vi "LET Transfer v2.vi"() -> ()   [LabVIEW 2010]
doc: "Cont(inuous) Acq(uire) & Chart (hw timed) demonstrates the hardware timed, non-buffered technique of data acquisition. The scan clock on the board controls acquisition timing. Acquired scans are read directly from the device's FIFO using AI Single Scan. \n\nThe acquisition is configured with no buffer, and the on-board scan clock started at the selected scan rate. In the first loop iteration, the newest (most recent) scan is read from the FIFO. In each subsequent loop iteration AI Single Scan is called to read the oldest scan from the FIFO. Then if a scan is missed because the acquisition does not keep up, an error message will be displayed, and the acquisition stopped. Each scan is plotted on the chart after it is read. \n\nA common reason to use non-buffered acquisition is that some kind of processing needs to be done for each data point. You will probably want to add more functions to the diagram to customize this VI for your application. The acquisition rate you can achieve depends on how much processing and display the VI must do. This VI calls a subVI named My Single-Scan Processing. Add whatever processing you need to this subVI, or replace it with one of your own. The data processing subVI also demonstrates how to use error clusters in your own subVIs, so they can be included in the error data flow chain.\n\nBefore running this VI, set the values of the controls on the front panel. Select Show Help Window from the Help menu to see a description of each control. If the values you select for all the controls are values you will usually use, select Make Current Values Default from the Operate menu and save the VI. Or, you may save individual control's default values by popping up on the control, selecting Data Operations, then selecting Make Current Value Default, and saving the VI."
uses:
  <instrlib>/agilent_b2900_series/Agilent B2900 Series/Public/Configure/Measurement/Configure Measurement (Current).vi
  <instrlib>/agilent_b2900_series/Agilent B2900 Series/Public/Configure/Measurement/Configure Measurement (Voltage).vi
  <vilib>/Utility/file.llb/Write To Spreadsheet File (DBL).vi
  <instrlib>/agilent_b2900_series/Agilent B2900 Series/Agilent B2900 Series.lvlib
panel:
  out "data matrix":dbl[][](array[numeric])
  out "Igs array 2":dbl[][](array[numeric])
  out "Vgs array 2":dbl[][](array[numeric])
  out "Vds array 2":dbl[][](array[numeric])
  out "Corrected PD current array 2":dbl[][](array[numeric])
  out "Ids array 2":dbl[][](array[numeric])
  out "corrected PD current array":dbl[](array[numeric])
  out "Vds array":dbl[](array[numeric])
  out "Ids array":dbl[](array[numeric])
  out "Vgs array":dbl[](array[numeric])
  out "Igs array":dbl[](array[numeric])
  in  "Tab Control":T1(tab)
  in  "keithley address":string="GPIB0::20::INSTR"
  in  "agilent address":refnum<visa-resource-name>="GPIB0::23::INSTR"
  in  "Initial Vgs (V)":sgl format="%.2f"
  in  "Vgs step (V)":sgl=1.0 format="%.2f"
  in  "Vgs delay time (ms)":sgl=10.0 format="%.2f"
  in  "Vgs delay after first value":sgl=10.0 caption="Vgs delay after first value (ms)" format="%.2f"
  in  "Final Vgs(V)":sgl=60.0 format="%.2f"
  in  "light emission ON/OFF":bool=TRUE
  in  "Vds step (V)":sgl=20.0 format="%.2f"
  in  "Final Vds (V)":sgl=60.0 format="%.2f"
  in  "Initial Vds (V)":sgl format="%.2f"
  in  "Vds hold time (ms)":i32=10
  in  "Compliance Voltage (channel 1)":dbl=60.0
  in  "Compliance Current (channel 2)":dbl=0.001
  in  "Compliance Voltage (channel 2)":dbl=60.0
  in  "Compliance Current (channel 1)":dbl=0.0001
  in  "keithley compliance limit":dbl(ring)=0.025 items=["25uA"=2.5e-05, "250uA"=0.00025, "2.5mA"=0.0025, "25mA"=0.025]
  in  "Loop":bool=TRUE
  in  "Auto Current NPLC (F: Disable)":bool
  in  "Auto Voltage NPLC(F: Disable)":bool
  in  "Current NPLC (0.1)":dbl=0.1
  in  "Voltage NPLC (0.1 PLC)":dbl=0.1
  in  "Current Auto Range Mode (0: Normal)":i32(ring) items=["Normal", "Resolution", "Speed"]
  in  "Voltage Auto Range Mode (0: Normal)":i32(ring) items=["Normal", "Resolution", "Speed"]
  in  "aperture time":dbl(ring)=-3.0 format="%.2f" items=["KE6485_VAL_RATE_FAST"=-1.0, "KE6485_VAL_RATE_MEDIUM"=-2.0, "KE6485_VAL_RATE_SLOW"=-3.0]
  in  "resolution (absolute)":dbl=0.0001 format="%^.2e"
  in  "Tab Control 2":enum32{"log scale", "linear scale"}(tab)
  out "Current Scan log":cluster{dbl[], dbl[]}(graph) caption="Current Scan"
  out "Current Scan log2":cluster{dbl[], dbl[]}(graph) caption="Current Scan"
  out "Current Scan linear":cluster{dbl[], dbl[]}(graph) caption="Current Scan"
  out "Current Scan linear 2":cluster{dbl[], dbl[]}(graph) caption="Current Scan"
  out "Applied Vgs":sgl caption="current VDS (V)" format="%.2f"
  out "Applied Vds":sgl caption="current VDS (V)" format="%.2f"
  out "Measured Ids":dbl format="%.2e"
  out "Measured Vds":dbl
  out "corrected PD current":dbl format="%^.2e"
  out "dark PD current (A)":dbl format="%^.2e"
  out "PD current":dbl format="%^.2e"
  out "Measured Igs":dbl
  out "Measured Vgs":dbl
  out "channel 2 status":bool
  out "channel 1 status":bool
  out "half  points":sgl
  out "Vgs points":sgl
  out "Vds points":sgl
  in  "Tab Control 3":enum32{"Log scale", "Linear scale"}(tab)
  out "?":cluster{dbl[], dbl[]}[](graph)
  out "?":cluster{dbl[], dbl[]}[](graph)
  out "?":cluster{dbl[], dbl[]}[](graph)
  out "?":cluster{dbl[], dbl[]}[](graph)
  in  "error in keithley":errorcluster
  out "keithley address out":refnum<k15>
  out "error out keithley":errorcluster
  out "error out agilent":errorcluster
  out "Agilent address out":refnum<visa-resource-name>
  # "LET Transfer v2"
  # "Gate Setting"
  # "Drain-source Setting"
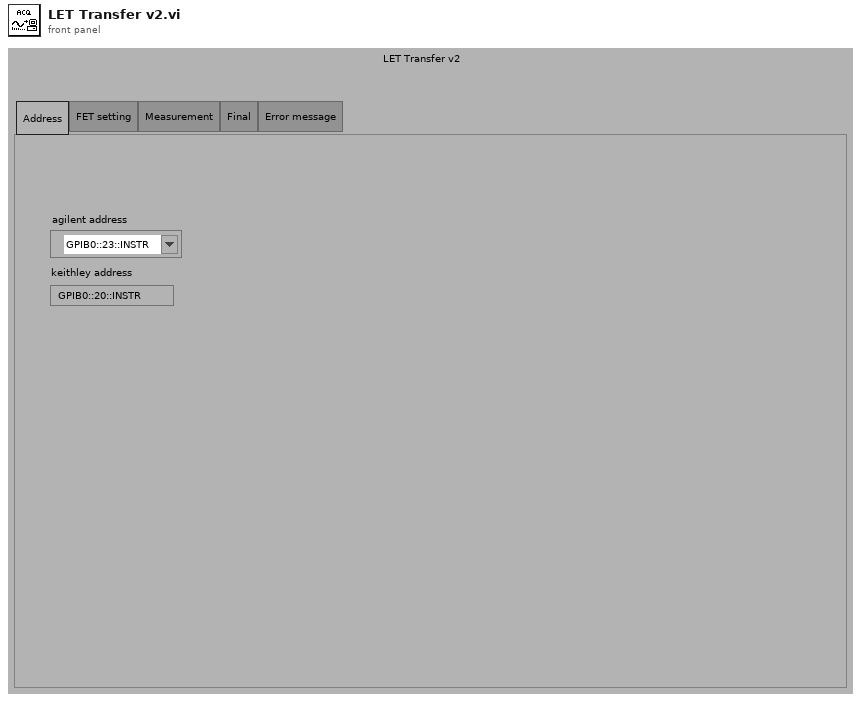
[diagram p1: front panel]
types:
  T1 = enum32{"Address", "FET setting", "Measurement", "Final", "Error message"}
  T2 = typedef "NI_Matrix.lvlib/RealMatrix.ctl" = dbl[][]
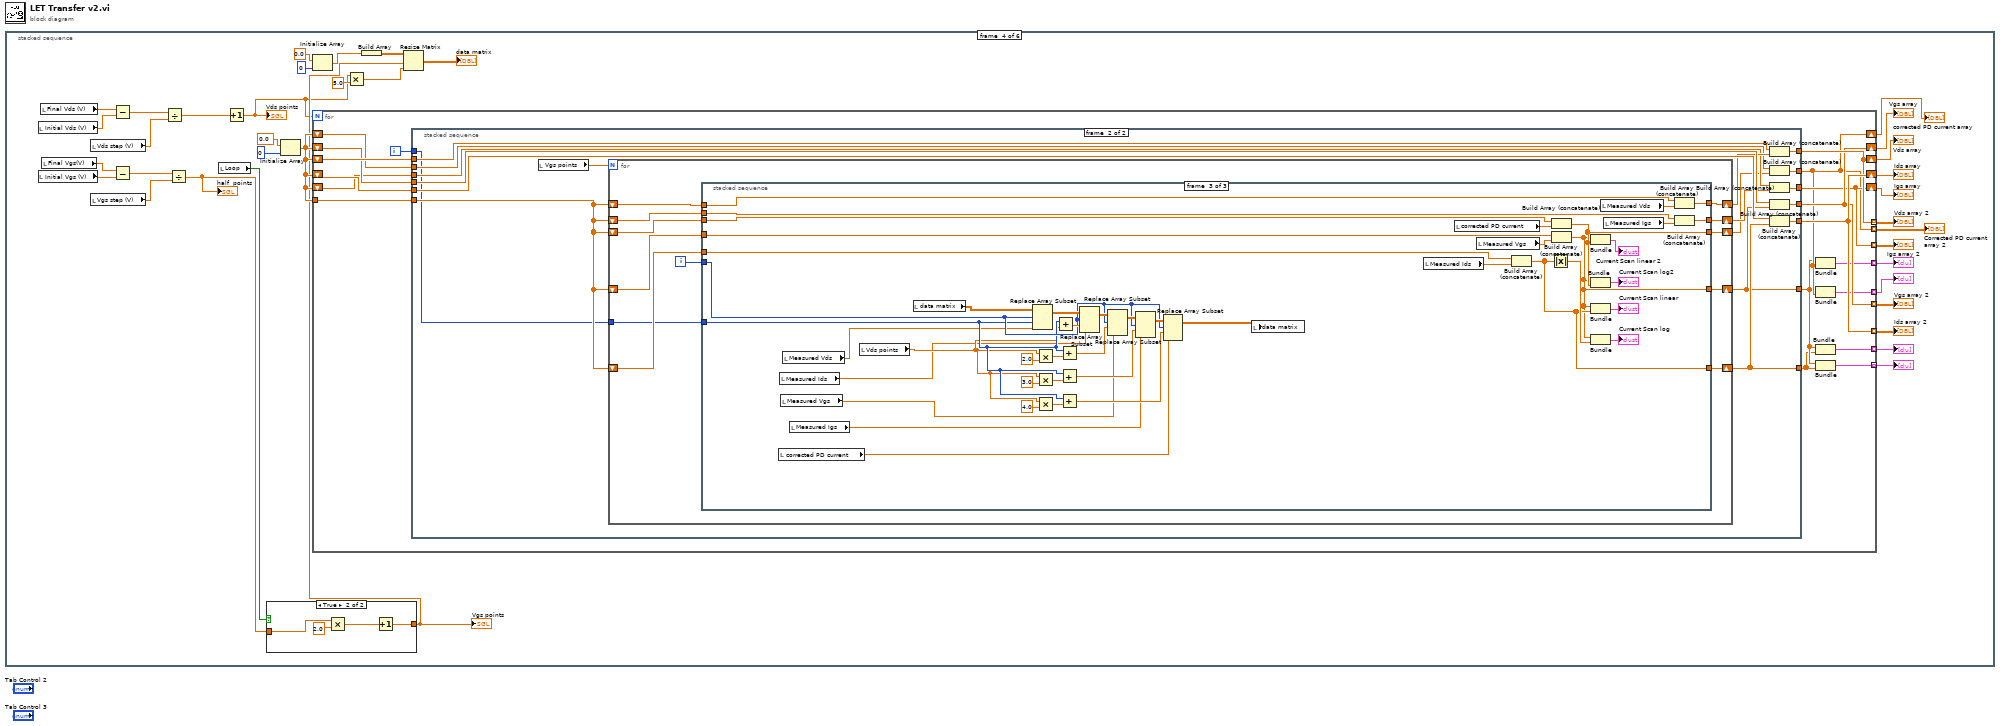
[diagram p0: block diagram]
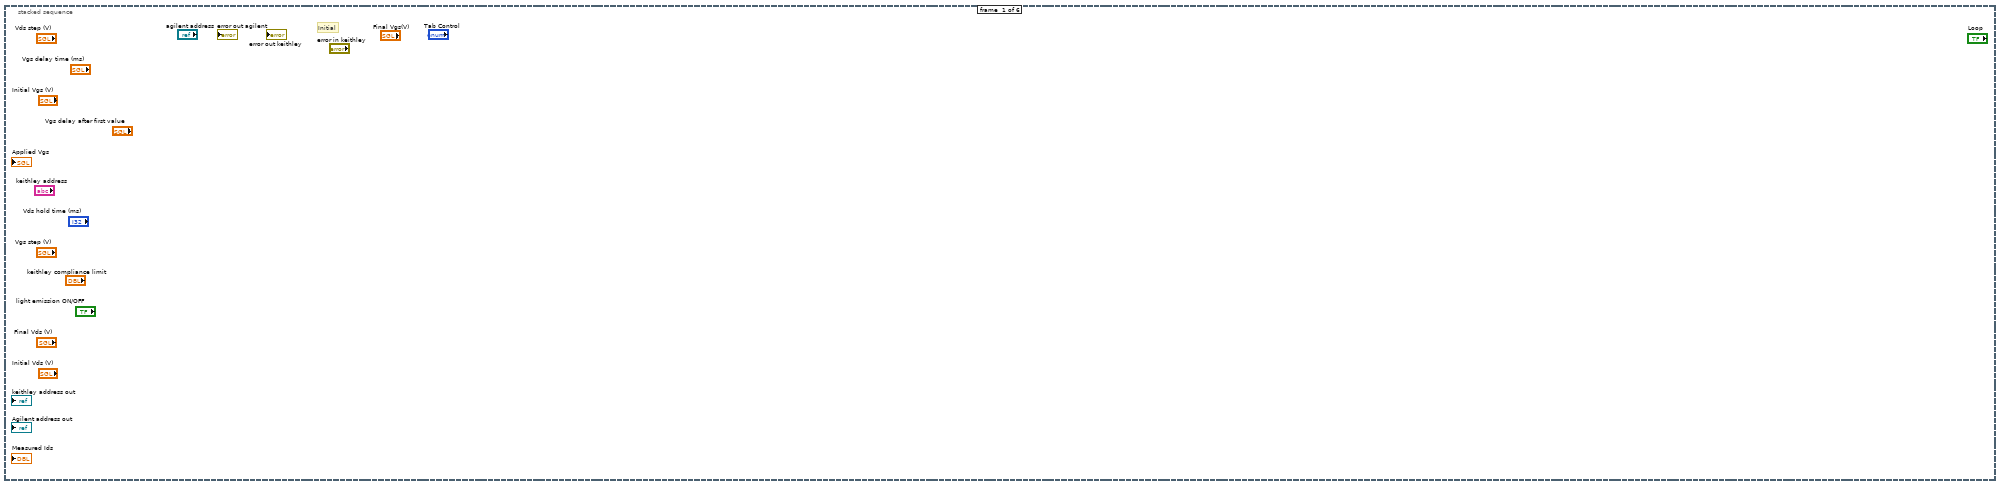
[diagram p2: hidden frame]
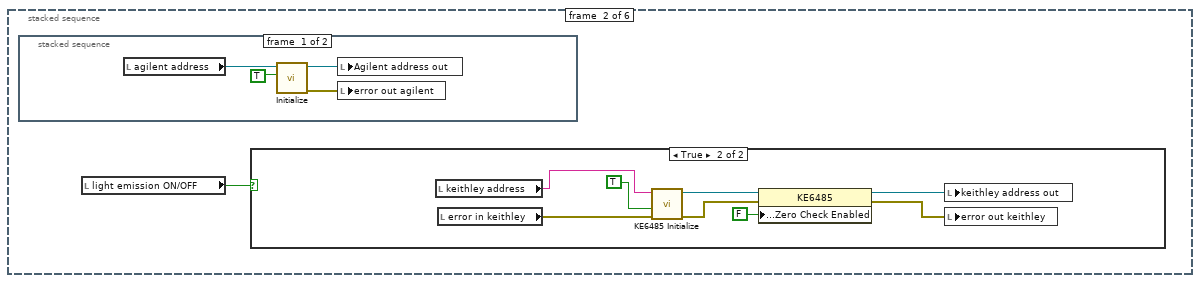
[diagram p3: hidden frame]
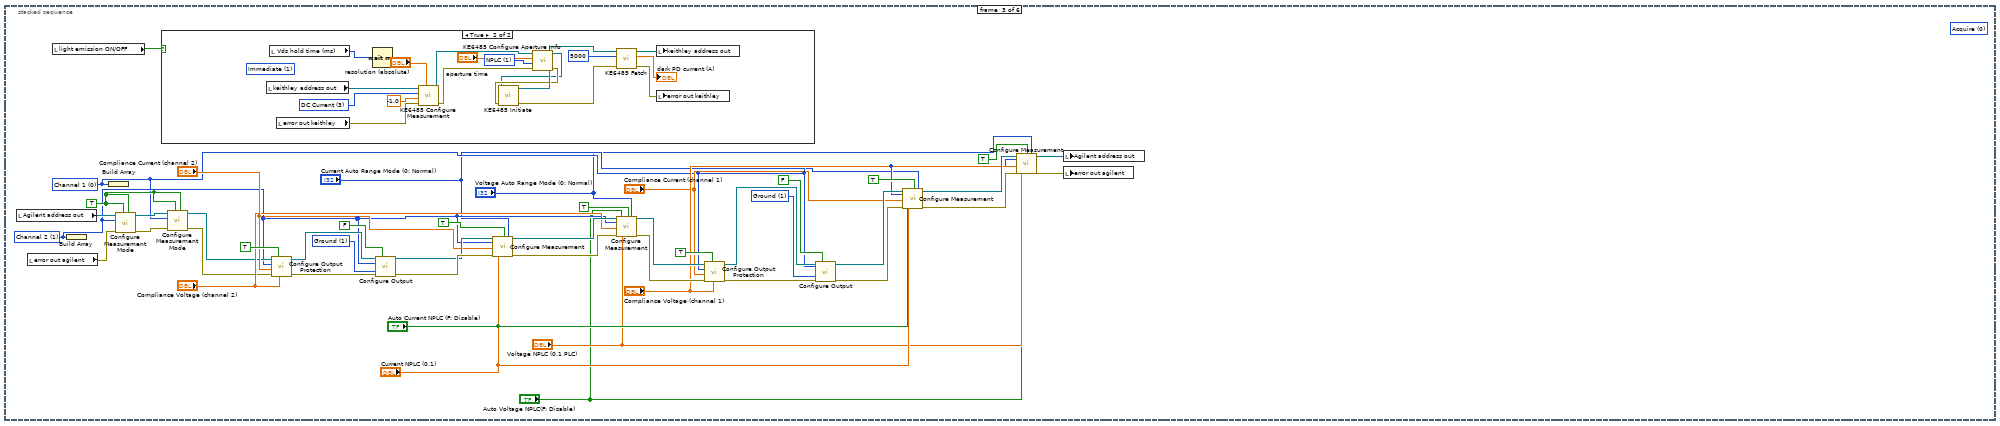
[diagram p6: hidden frame]
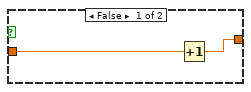
[diagram p8: hidden frame]
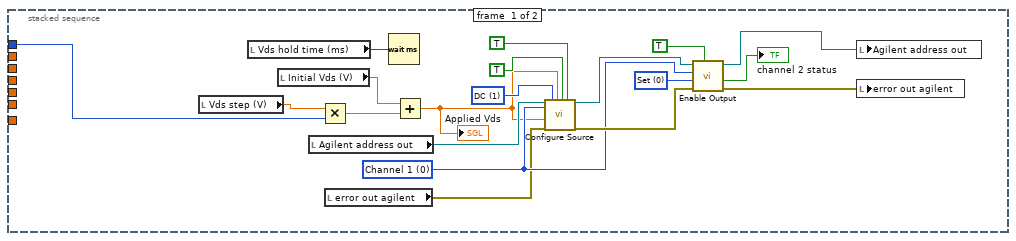
[diagram p9: hidden frame]
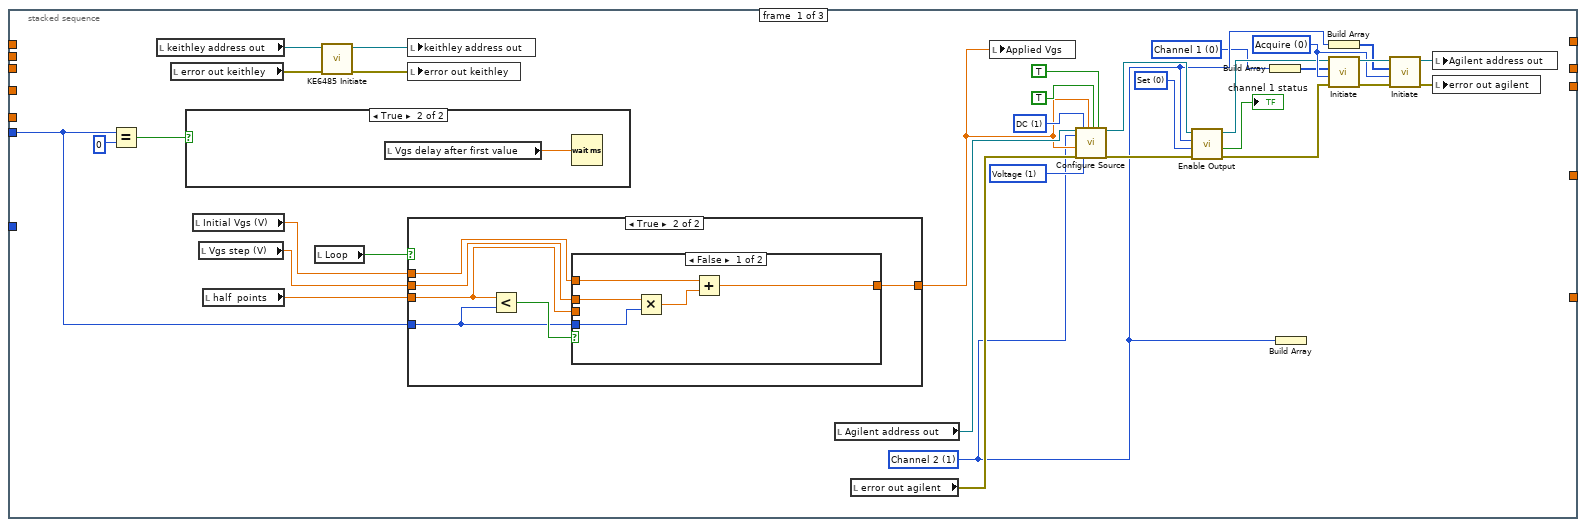
[diagram p10: hidden frame]
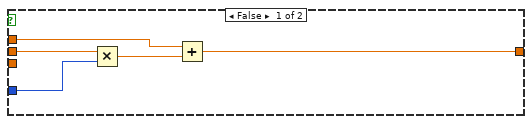
[diagram p11: hidden frame]
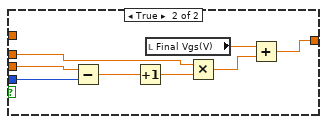
[diagram p12: hidden frame]
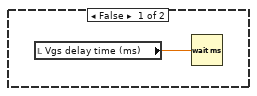
[diagram p13: hidden frame]
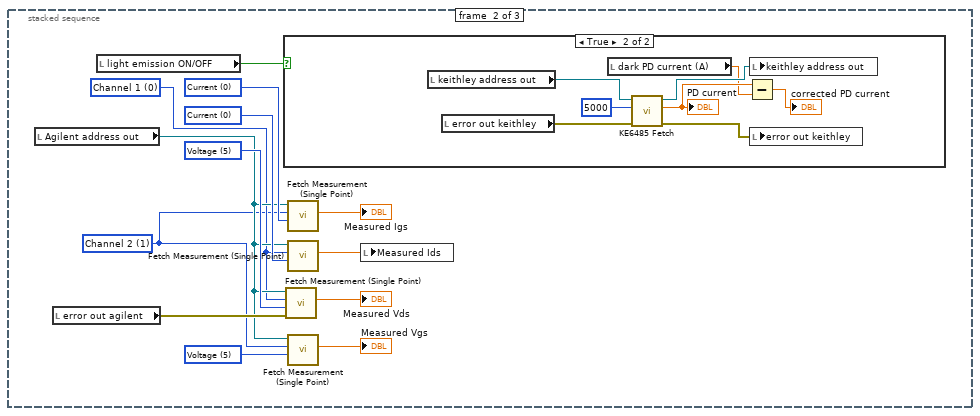
[diagram p14: hidden frame]
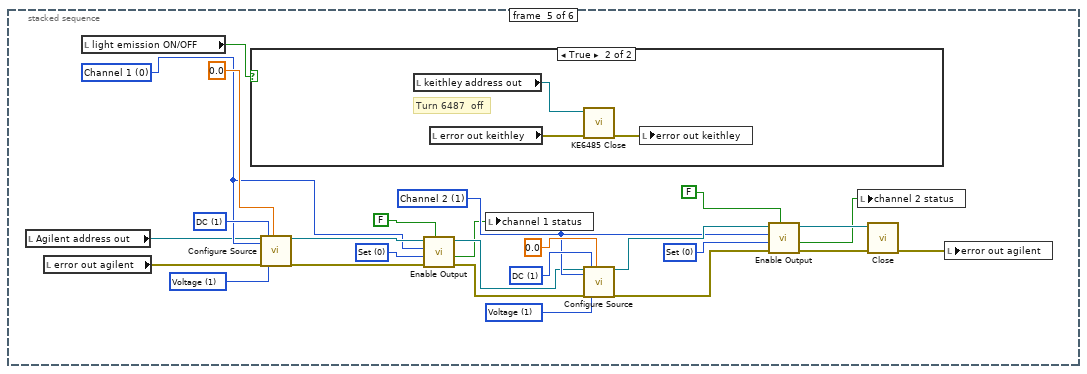
[diagram p16: hidden frame]
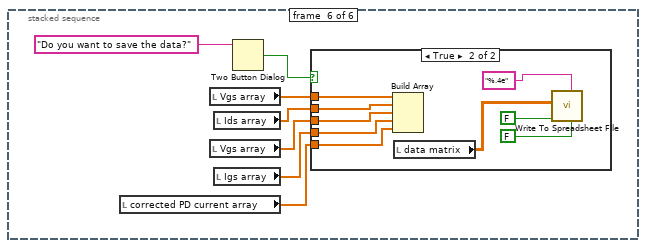
[diagram p18: hidden frame]
diagram:
  n1 = stacked-sequence {
    frame #0 {
      # "Initial"
    }
    frame #1 {
      n2 = stacked-sequence {
        frame #0 {
          n3 = local read "agilent address"() -> (w2:refnum<visa-resource-name>)
          n4 = call <instrlib>:"Initialize.vi"("ID Query (True)"=TRUE, "VISA resource name"=w2) -> ("error out"=w3:errorcluster, "VISA resource name out"=w4:refnum<visa-resource-name>)  [unwired: 8 in]
          n5 = local write "Agilent address out"(w4) -> ()
          n6 = local write "error out agilent"(w3) -> ()
        }
        frame #1 {
        }
      }
      n7 = local read "light emission ON/OFF"() -> (w1:bool)
      n8 = case shown="True" w1 {
        frame False {
        }
        frame True {
          n9 = local read "keithley address"() -> (w12:string)
          n10 = local read "error in keithley"() -> (w13:errorcluster)
          n11 = call <instrlib>:"KE6485 Initialize.vi"("error in (no error)"=w13, "reset device"=TRUE, "resource name"=w12) -> ("error out"=w10:errorcluster, "instrument handle out"=w9:refnum<k15>)  [unwired: 1 in, 6 out]
          n12 = property class="KE6485"(reference=w9, error in=w10, "System Settings:Zero Check Enabled"=FALSE) -> (reference out=w8:refnum<k15>, error out=w7:errorcluster)
          n13 = local write "keithley address out"(w8) -> ()
          n14 = local write "error out keithley"(w7) -> ()
        }
      }
    }
    frame #2 {
      (unwired) 0 items=["Acquire", "Transient", "Both"] ("Device Action (2: Both)")
      w30 = TRUE ("Enable Voltage Measurement (T: Enable)")
      w42 = 1 items=["Float", "Ground"] ("Low Terminal State (1: Ground)")
      w22 = 0 items=["Channel 1", "Channel 2"] ("Channel (0: Channel 1)")
      w52 = 1 items=["Float", "Ground"] ("Low Terminal State (1: Ground)")
      w23 = 1 items=["Channel 1", "Channel 2"] ("Channel (0: Channel 1)")
      n15 = local read "Agilent address out"() -> (w25:refnum<visa-resource-name>)
      n16 = local read "error out agilent"() -> (w27:errorcluster)
      n17 = local read "light emission ON/OFF"() -> (w59:bool)
      n18 = Build Array(w23) -> ()  [unwired: 1 out]
      n19 = Build Array(w22) -> ()  [unwired: 1 out]
      n20 = call <instrlib>:"Configure Measurement Mode.vi"("Enable Current Measurement (T: Enable)"=w30, "Enable Voltage Measurement (T: Enable)"=w30, "error in (no error)"=w27, "Channel (0: Channel 1)"=w23, "VISA resource name"=w25) -> ("error out"=w28:errorcluster, "VISA resource name out"=w29:refnum<visa-resource-name>)  [unwired: 5 in]
      n21 = case shown="True" w59 {
        frame False {
        }
        frame True {
          w66 = 1 items=["NPLC"=1] ("aperture time unit")
          (unwired) 1 items=["Immediate"=1, "Interval"=10, "Trigger Link 1"=1001, "Trigger Link 2"=1002, "Trigger Link 3"=1003, "Trigger Link 4"=1004, "Trigger Link 5"=1005, "Trigger Link 6"=1006] ("sample trigger")
          w75 = 3 items=["DC Volts"=1, "DC Current"=3, "2 Wire Resistance"=5, "Charge"=1004] ("measurement function")
          n22 = local read "keithley address out"() -> (w70:refnum<k15>)
          n23 = local read "Vds hold time (ms)"() -> (w77:i32)
          n24 = local read "error out keithley"() -> (w69:errorcluster)
          n25 = Wait (ms)(milliseconds to wait=w77) -> ()  [unwired: 1 out]
          n26 = call <instrlib>:"KE6485 Configure Measurement.vi"("resolution (absolute)"="resolution (absolute)", "error in (no error)"=w69, "range"=-1.0, "measurement function"=w75, "instrument handle"=w70) -> ("error out"=w65:errorcluster, "instrument handle out"=w64:refnum<k15>)  [unwired: 5 in]
          n27 = call <instrlib>:"KE6485 Configure Aperture Info.vi"("error in (no error)"=w65, "aperture time unit"=w66, "aperture time"="aperture time", "instrument handle"=w64) -> ("error out"=w63:errorcluster, "instrument handle out"=w62:refnum<k15>)  [unwired: 6 in]
          n28 = call <instrlib>:"KE6485 Initiate.vi"("error in (no error)"=w63, "instrument handle"=w62) -> ("error out"=w67:errorcluster, "instrument handle out"=w68:refnum<k15>)  [unwired: 8 in]
          n29 = call <instrlib>:"KE6485 Fetch.vi"("error in (no error)"=w67, "maximum time (ms)"=5000, "instrument handle"=w68) -> ("error out"=w72:errorcluster, "reading"=→"dark PD current (A)":dbl, "instrument handle out"=w71:refnum<k15>)  [unwired: 6 in]
          n30 = local write "keithley address out"(w71) -> ()
          n31 = local write "error out keithley"(w72) -> ()
        }
      }
      n32 = call <instrlib>:"Configure Measurement Mode.vi"("Enable Current Measurement (T: Enable)"=w30, "Enable Voltage Measurement (T: Enable)"=w30, "error in (no error)"=w28, "Channel (0: Channel 1)"=w22, "VISA resource name"=w29) -> ("error out"=w26:errorcluster, "VISA resource name out"=w24:refnum<visa-resource-name>)  [unwired: 5 in]
      n33 = call <instrlib>:"Configure Output Protection.vi"("Compliance Voltage (2 V)"="Compliance Voltage (channel 2)", "Enable Output Protection (T: Enable)"=TRUE, "error in (no error)"=w26, "Compliance Current (0.0001 A)"="Compliance Current (channel 2)", "Channel (0: Channel 1)"=w23, "VISA resource name"=w24) -> ("error out"=w54:errorcluster, "VISA resource name out"=w53:refnum<visa-resource-name>)  [unwired: 4 in]
      n34 = call <instrlib>:"Configure Output.vi"("VISA resource name"=w53, "Auto Output-Off (F: Disable)"=FALSE, "Channel (0: Channel 1)"=w23, "Low Terminal State (1: Ground)"=w52, "error in (no error)"=w54) -> ("VISA resource name out"=w50:refnum<visa-resource-name>, "error out"=w51:errorcluster)  [unwired: 9 in]
      n35 = call-poly <instrlib>:"Configure Measurement.vi"("VISA resource name"=w50, "Channel (0: Channel 1)"=w23, "Current Range (0.0001 A)"="Compliance Current (channel 2)", "error in (no error)"=w51, "Auto Current NPLC (F: Disable)"="Auto Current NPLC (F: Disable)", "Current NPLC (0.1)"="Current NPLC (0.1)", "Current Auto Range (T: Enable)"=TRUE, "Current Auto Range Mode (0: Normal)"="Current Auto Range Mode (0: Normal)") -> ("VISA resource name out"=w58:refnum<visa-resource-name>, "error out"=w57:errorcluster)  [unwired: 10 in]
      n36 = call-poly <instrlib>:"Configure Measurement.vi"("VISA resource name"=w58, "Channel (0: Channel 1)"=w23, "Voltage Range (2 V)"="Compliance Voltage (channel 2)", "error in (no error)"=w57, "Auto Voltage NPLC(F: Disable)"="Auto Voltage NPLC(F: Disable)", "Voltage NPLC (0.1 PLC)"="Voltage NPLC (0.1 PLC)", "Voltage Auto Range (T: Enable)"=TRUE, "Voltage Auto Range Mode (0: Normal)"="Voltage Auto Range Mode (0: Normal)") -> ("VISA resource name out"=w38:refnum<visa-resource-name>, "error out"=w37:errorcluster)  [unwired: 10 in]
      n37 = call <instrlib>:"Configure Output Protection.vi"("Compliance Voltage (2 V)"="Compliance Voltage (channel 1)", "Enable Output Protection (T: Enable)"=TRUE, "error in (no error)"=w37, "Compliance Current (0.0001 A)"="Compliance Current (channel 1)", "Channel (0: Channel 1)"=w22, "VISA resource name"=w38) -> ("error out"=w44:errorcluster, "VISA resource name out"=w43:refnum<visa-resource-name>)  [unwired: 4 in]
      n38 = call <instrlib>:"Configure Output.vi"("VISA resource name"=w43, "Auto Output-Off (F: Disable)"=FALSE, "Channel (0: Channel 1)"=w22, "Low Terminal State (1: Ground)"=w42, "error in (no error)"=w44) -> ("VISA resource name out"=w40:refnum<visa-resource-name>, "error out"=w41:errorcluster)  [unwired: 9 in]
      n39 = call-poly <instrlib>:"Configure Measurement.vi"("VISA resource name"=w40, "Channel (0: Channel 1)"=w22, "Current Range (0.0001 A)"="Compliance Current (channel 1)", "error in (no error)"=w41, "Auto Current NPLC (F: Disable)"="Auto Current NPLC (F: Disable)", "Current NPLC (0.1)"="Current NPLC (0.1)", "Current Auto Range (T: Enable)"=TRUE, "Current Auto Range Mode (0: Normal)"="Current Auto Range Mode (0: Normal)") -> ("VISA resource name out"=w48:refnum<visa-resource-name>, "error out"=w47:errorcluster)  [unwired: 10 in]
      n40 = call-poly <instrlib>:"Configure Measurement.vi"("VISA resource name"=w48, "Channel (0: Channel 1)"=w22, "Voltage Range (2 V)"="Compliance Voltage (channel 1)", "error in (no error)"=w47, "Auto Voltage NPLC(F: Disable)"="Auto Voltage NPLC(F: Disable)", "Voltage NPLC (0.1 PLC)"="Voltage NPLC (0.1 PLC)", "Voltage Auto Range (T: Enable)"=TRUE, "Voltage Auto Range Mode (0: Normal)"="Voltage Auto Range Mode (0: Normal)") -> ("VISA resource name out"=w21:refnum<visa-resource-name>, "error out"=w20:errorcluster)  [unwired: 10 in]
      n41 = local write "Agilent address out"(w21) -> ()
      n42 = local write "error out agilent"(w20) -> ()
    }
    frame #3 {
      n43 = local read "Initial Vds (V)"() -> (w103:sgl)
      n44 = local read "Initial Vgs (V)"() -> (w106:sgl)
      n45 = local read "Final Vds (V)"() -> (w102:sgl)
      n46 = local read "Final Vgs(V)"() -> (w105:sgl)
      n47 = local read "Vds step (V)"() -> (w104:sgl)
      n48 = local read "Vgs step (V)"() -> (w107:sgl)
      n49 = Subtract(x=w102, y=w103) -> (x-y=w100:sgl)
      n50 = Subtract(x=w105, y=w106) -> (x-y=w114:sgl)
      n51 = Divide(x=w100, y=w104) -> (x/y=w101:sgl)
      n52 = Divide(x=w114, y=w107) -> (x/y=w98:sgl)
      "half  points" <- w98
      n53 = local read "Loop"() -> (w99:bool)
      n54 = Increment(x=w101) -> (x+1=w78:sgl)
      "Vds points" <- w78
      n55 = case shown="True" w99 {
        tunnel: w98 -> [w116 w120]
        tunnel: [w115 w118] -> w81
        frame False {
          n56 = Increment(x=w116) -> (x+1=w115:sgl)
        }
        frame True {
          n57 = Multiply(x=w120, y=sgl 2.0) -> (x*y=w117:sgl)
          n58 = Increment(x=w117) -> (x+1=w118:sgl)
        }
      }
      "Vgs points" <- w81
      n59 = Initialize Array(0.0, 0) -> (w95:dbl[])
      n60 = Initialize Array(0.0 ("element"), 0 ("dimension size")) -> (w84:dbl[])
      n61 = for {
        N: w78 -> [_]
        shift-right: [w129] -> w110
        shift-left: w95 -> [w137]
        shift-right: [w130] -> w111
        shift-left: w95 -> [w136]
        shift-right: [w128] -> w109
        shift-left: w95 -> [w135]
        tunnel: [w134] -> w108 mode=indexing
        shift-right: [w127] -> w97
        shift-left: w95 -> [w133]
        shift-right: [w125] -> w96
        shift-left: w95 -> [w132]
        tunnel: w95 -> [w131]
        tunnel: [w130] -> w94 mode=indexing
        tunnel: [w125] -> w93 mode=indexing
        tunnel: [w129] -> w92 mode=indexing
        tunnel: [w128] -> w91 mode=indexing
        tunnel: [w127] -> w90 mode=indexing
        tunnel: [w126] -> w89 mode=indexing
        tunnel: [w124] -> w88 mode=indexing
        tunnel: [w121] -> w87 mode=indexing
        i -> [w138]
        n62 = stacked-sequence {
          tunnel: w138 -> [w153 w158]
          tunnel: w137 -> [_ w175]
          tunnel: w136 -> [_ w174]
          tunnel: [_ w170] -> w129
          tunnel: [_ w173] -> w130
          tunnel: w135 -> [_ w172]
          tunnel: [_ w171] -> w128
          tunnel: [_ w159] -> w123
          tunnel: [_ w168] -> w122
          tunnel: w133 -> [_ w167]
          tunnel: [_ w166] -> w127
          tunnel: [_ w164] -> w125
          tunnel: w132 -> [_ w162]
          tunnel: w131 -> [_ w160]
          frame #0 {
            w146 = 0 items=["Set", "Get"] ("Operation (0: Set)")
            w147 = 0 items=["Channel 1", "Channel 2"] ("Channel (0: Channel 1)")
            w150 = 1 items=["Pulse", "DC"] ("Source Shape (1: DC)")
            n63 = local read "Vds step (V)"() -> (w157:sgl)
            n64 = local read "Vds hold time (ms)"() -> (w155:i32)
            n65 = local read "Initial Vds (V)"() -> (w156:sgl)
            n66 = local read "Agilent address out"() -> (w143:refnum<visa-resource-name>)
            n67 = Multiply(x=w157, y=w153) -> (x*y=w154:sgl)
            n68 = local read "error out agilent"() -> (w142:errorcluster)
            n69 = Wait (ms)(milliseconds to wait=w155) -> ()  [unwired: 1 out]
            n70 = Add(x=w156, y=w154) -> (x+y=w139:sgl)
            "Applied Vds" <- w139
            n71 = call <instrlib>:"Configure Source.vi"("VISA resource name"=w143, "Channel (0: Channel 1)"=w147, "Source Range (2)"=w139, "error in (no error)"=w142, "Source Shape (1: DC)"=w150, "Output Level (0)"=w139, "Source Auto Range (T: Enable)"=TRUE, "Enable Continuous Output (T: Enable)"=TRUE) -> ("VISA resource name out"=w152:refnum<visa-resource-name>, "error out"=w151:errorcluster)  [unwired: 10 in]
            n72 = call <instrlib>:"Enable Output.vi"("Enable Output (T: Enable)"=TRUE, "error in (no error)"=w151, "Operation (0: Set)"=w146, "Channel (0: Channel 1)"=w147, "VISA resource name"=w152) -> ("error out"=w141:errorcluster, "Output Enabled?"=→"channel 2 status":bool, "VISA resource name out"=w140:refnum<visa-resource-name>)  [unwired: 4 in]
            n73 = local write "Agilent address out"(w140) -> ()
            n74 = local write "error out agilent"(w141) -> ()
          }
          frame #1 {
            n75 = local read "Vgs points"() -> (w161:sgl)
            n76 = for {
              N: w161 -> [_]
              shift-right: [w178] -> w168
              shift-left: w160 -> [w177]
              shift-right: [w180] -> w169
              shift-left: w160 -> [w179]
              shift-right: [w184] -> w159
              shift-left: w160 -> [w183]
              shift-right: [w182] -> w165
              shift-left: w160 -> [w181]
              shift-right: [w185] -> w163
              shift-left: w160 -> [w186]
              tunnel: w158 -> [w176]
              i -> [w187]
              n77 = stacked-sequence {
                tunnel: w187 -> [w207 _ w276]
                tunnel: w186 -> [_ _ w310]
                tunnel: [_ _ w295] -> w185
                tunnel: [_ _ w292] -> w184
                tunnel: w183 -> [_ _ w308]
                tunnel: [_ _ w294] -> w182
                tunnel: w181 -> [_ _ w306]
                tunnel: [_ _ w299] -> w180
                tunnel: w179 -> [_ _ w303]
                tunnel: [_ _ w293] -> w178
                tunnel: w177 -> [_ _ w301]
                tunnel: w176 -> [_ _ w275]
                frame #0 {
                  w200 = 0 items=["Acquire", "Transient", "Both"] ("Device Action (2: Both)")
                  w192 = 0 items=["Channel 1", "Channel 2"] ("Channel (0: Channel 1)")
                  w209 = 1 items=["Current", "Voltage"] ("Source Mode (1: Voltage)")
                  w212 = 1 items=["Pulse", "DC"] ("Source Shape (1: DC)")
                  w193 = 1 items=["Channel 1", "Channel 2"] ("Channel (0: Channel 1)")
                  w216 = 0 items=["Set", "Get"] ("Operation (0: Set)")
                  n78 = Equal?(x=w207, y=0) -> (x = y?=w219:bool)
                  n79 = local read "keithley address out"() -> (w189:refnum<k15>)
                  n80 = local read "error out keithley"() -> (w188:errorcluster)
                  n81 = case shown="True" w219 {
                    frame False {
                      n82 = local read "Vgs delay time (ms)"() -> (w245:sgl)
                      n83 = Wait (ms)(milliseconds to wait=w245) -> ()  [unwired: 1 out]
                    }
                    frame True {
                      n84 = local read "Vgs delay after first value"() -> (w246:sgl)
                      n85 = Wait (ms)(milliseconds to wait=w246) -> ()  [unwired: 1 out]
                    }
                  }
                  n86 = local read "Initial Vgs (V)"() -> (w208:sgl)
                  n87 = local read "Vgs step (V)"() -> (w206:sgl)
                  n88 = local read "half  points"() -> (w204:sgl)
                  n89 = local read "Loop"() -> (w205:bool)
                  n90 = call <instrlib>:"KE6485 Initiate.vi"("error in (no error)"=w188, "instrument handle"=w189) -> ("error out"=w191:errorcluster, "instrument handle out"=w190:refnum<k15>)  [unwired: 8 in]
                  n91 = local write "keithley address out"(w190) -> ()
                  n92 = local write "error out keithley"(w191) -> ()
                  n93 = case shown="True" w205 {
                    tunnel: [w224 w230] -> w203
                    tunnel: w207 -> [w223 w227]
                    tunnel: w208 -> [w222 w229]
                    tunnel: w206 -> [w221 w228]
                    tunnel: w204 -> [_ w226]
                    frame False {
                      n94 = Multiply(x=w221, y=w223) -> (x*y=w225:sgl)
                      n95 = Add(x=w222, y=w225) -> (x+y=w224:sgl)
                    }
                    frame True {
                      n96 = Less?(x=w226, y=w227) -> (x < y?=w231:bool)
                      n97 = case shown="False" w231 {
                        tunnel: [w235 w244] -> w230
                        tunnel: w229 -> [w234 _]
                        tunnel: w227 -> [w233 w241]
                        tunnel: w228 -> [w232 w242]
                        tunnel: w226 -> [_ w240]
                        frame False {
                          n98 = Multiply(x=w232, y=w233) -> (x*y=w236:sgl)
                          n99 = Add(x=w234, y=w236) -> (x+y=w235:sgl)
                        }
                        frame True {
                          n100 = Subtract(x=w240, y=w241) -> (x-y=w238:sgl)
                          n101 = Increment(x=w238) -> (x+1=w237:sgl)
                          n102 = local read "Final Vgs(V)"() -> (w239:sgl)
                          n103 = Multiply(x=w242, y=w237) -> (x*y=w243:sgl)
                          n104 = Add(x=w239, y=w243) -> (x+y=w244:sgl)
                        }
                      }
                    }
                  }
                  n105 = local read "Agilent address out"() -> (w214:refnum<visa-resource-name>)
                  n106 = local read "error out agilent"() -> (w213:errorcluster)
                  n107 = local write "Applied Vgs"(w203) -> ()
                  n108 = call <instrlib>:"Configure Source.vi"("VISA resource name"=w214, "Channel (0: Channel 1)"=w193, "Source Range (2)"=w203, "error in (no error)"=w213, "Source Shape (1: DC)"=w212, "Source Mode (1: Voltage)"=w209, "Output Level (0)"=w203, "Source Auto Range (T: Enable)"=TRUE, "Enable Continuous Output (T: Enable)"=TRUE) -> ("VISA resource name out"=w218:refnum<visa-resource-name>, "error out"=w217:errorcluster)  [unwired: 9 in]
                  n109 = call <instrlib>:"Enable Output.vi"("error in (no error)"=w217, "Operation (0: Set)"=w216, "Channel (0: Channel 1)"=w193, "VISA resource name"=w218) -> ("error out"=w196:errorcluster, "Output Enabled?"=→"channel 1 status":bool, "VISA resource name out"=w197:refnum<visa-resource-name>)  [unwired: 5 in]
                  n110 = Build Array(w192) -> (w199:i32[])
                  n111 = Build Array(w193) -> ()  [unwired: 1 out]
                  n112 = Build Array(w193) -> (w198:i32[])
                  n113 = call <instrlib>:"Initiate.vi"("error in (no error)"=w196, "Device Action (2: Both)"=w200, "Channel List ({Channel1})"=w199, "VISA resource name"=w197) -> ("error out"=w202:errorcluster, "VISA resource name out"=w201:refnum<visa-resource-name>)  [unwired: 6 in]
                  n114 = call <instrlib>:"Initiate.vi"("error in (no error)"=w202, "Device Action (2: Both)"=w200, "Channel List ({Channel1})"=w198, "VISA resource name"=w201) -> ("error out"=w195:errorcluster, "VISA resource name out"=w194:refnum<visa-resource-name>)  [unwired: 6 in]
                  n115 = local write "Agilent address out"(w194) -> ()
                  n116 = local write "error out agilent"(w195) -> ()
                }
                frame #1 {
                  w248 = 1 items=["Channel 1", "Channel 2"] ("Channel (0: Channel 1)")
                  w249 = 0 items=["Channel 1", "Channel 2"] ("Channel (0: Channel 1)")
                  w254 = 0 items=["Current", "Resistance", "Source Output Setting", "Status", "Time", "Voltage"] ("Data Mode (5: Voltage)")
                  w255 = 5 items=["Current", "Resistance", "Source Output Setting", "Status", "Time", "Voltage"] ("Data Mode (5: Voltage)")
                  w257 = 0 items=["Current", "Resistance", "Source Output Setting", "Status", "Time", "Voltage"] ("Data Mode (5: Voltage)")
                  w259 = 5 items=["Current", "Resistance", "Source Output Setting", "Status", "Time", "Voltage"] ("Data Mode (5: Voltage)")
                  n117 = local read "Agilent address out"() -> (w250:refnum<visa-resource-name>)
                  n118 = local read "error out agilent"() -> (w251:errorcluster)
                  n119 = local read "light emission ON/OFF"() -> (w247:bool)
                  n120 = case shown="True" w247 {
                    frame False {
                    }
                    frame True {
                      n121 = local read "keithley address out"() -> (w261:refnum<k15>)
                      n122 = local read "error out keithley"() -> (w260:errorcluster)
                      n123 = local read "dark PD current (A)"() -> (w262:dbl)
                      n124 = call <instrlib>:"KE6485 Fetch.vi"("error in (no error)"=w260, "maximum time (ms)"=5000, "instrument handle"=w261) -> ("error out"=w266:errorcluster, "reading"=w263:dbl, "instrument handle out"=w265:refnum<k15>)  [unwired: 6 in]
                      "PD current" <- w263
                      n125 = Subtract(x=w263, y=w262) -> (x-y=→"corrected PD current":dbl)
                      n126 = local write "keithley address out"(w265) -> ()
                      n127 = local write "error out keithley"(w266) -> ()
                    }
                  }
                  n128 = call <instrlib>:"Fetch Measurement (Single Point).vi"("error in (no error)"=w251, "Data Mode (5: Voltage)"=w259, "Channel (0: Channel 1)"=w249, "VISA resource name"=w250) -> ("Measurement"=→"Measured Vds":dbl)  [unwired: 5 in, 2 out]
                  n129 = call <instrlib>:"Fetch Measurement (Single Point).vi"("Data Mode (5: Voltage)"=w254, "Channel (0: Channel 1)"=w248, "VISA resource name"=w250) -> ("Measurement"=→"Measured Igs":dbl)  [unwired: 6 in, 2 out]
                  n130 = call <instrlib>:"Fetch Measurement (Single Point).vi"("Data Mode (5: Voltage)"=w257, "Channel (0: Channel 1)"=w249, "VISA resource name"=w250) -> ("Measurement"=w256:dbl)  [unwired: 6 in, 2 out]
                  n131 = call <instrlib>:"Fetch Measurement (Single Point).vi"("Data Mode (5: Voltage)"=w255, "Channel (0: Channel 1)"=w248, "VISA resource name"=w250) -> ("Measurement"=→"Measured Vgs":dbl)  [unwired: 6 in, 2 out]
                  n132 = local write "Measured Ids"(w256) -> ()
                }
                frame #2 {
                  n133 = local read "corrected PD current"() -> (w273:dbl)
                  n134 = local read "Measured Ids"() -> (w270:dbl)
                  n135 = local read "Measured Vgs"() -> (w271:dbl)
                  n136 = local read "Measured Vds"() -> (w269:dbl)
                  n137 = local read "Measured Igs"() -> (w272:dbl)
                  n138 = local read "Vds points"() -> (w274:sgl)
                  n139 = local read "data matrix"() -> (w277:dbl[][])
                  n140 = Replace Array Subset(array=w277, new element=w269, index (row)=w276, index (col)=w275) -> (w291:T2)
                  n141 = Multiply(x=w274, y=sgl 2.0) -> (x*y=w287:sgl)
                  n142 = Multiply(x=w274, y=sgl 3.0) -> (x*y=w284:sgl)
                  n143 = Multiply(x=w274, y=sgl 4.0) -> (x*y=w280:sgl)
                  n144 = Add(x=w275, y=w274) -> (x+y=w290:sgl)
                  n145 = Add(x=w275, y=w287) -> (x+y=w288:sgl)
                  n146 = Add(x=w275, y=w284) -> (x+y=w282:sgl)
                  n147 = Add(x=w275, y=w280) -> (x+y=w278:sgl)
                  n148 = Replace Array Subset(array=w291, new element=w270, index (row)=w276, index (col)=w290) -> (w289:T2)
                  n149 = Replace Array Subset(array=w289, new element=w271, index (row)=w276, index (col)=w288) -> (w285:T2)
                  n150 = Replace Array Subset(array=w285, new element=w272, index (row)=w276, index (col)=w282) -> (w281:T2)
                  n151 = Replace Array Subset(array=w281, new element=w273, index (row)=w276, index (col)=w278) -> (w268:T2)
                  n152 = local write "data matrix"(w268) -> ()
                  n153 = local read "Measured Ids"() -> (w302:dbl)
                  n154 = local read "corrected PD current"() -> (w311:dbl)
                  n155 = local read "Measured Vgs"() -> (w309:dbl)
                  n156 = Build Array (concatenate)(w301, w302) -> (w293:dbl[])
                  n157 = Absolute Value(x=w293) -> (abs(x)=w298:dbl[])
                  n158 = Build Array (concatenate)(w310, w311) -> (w295:dbl[])
                  n159 = Build Array (concatenate)(w308, w309) -> (w292:dbl[])
                  n160 = Bundle(w292, w295) -> (→"Current Scan linear 2":cluster{dbl[], dbl[]})  [unwired: 1 out]
                  n161 = Bundle(w292, w295) -> (→"Current Scan log2":cluster{dbl[], dbl[]})  [unwired: 1 out]
                  n162 = Bundle(w292, w293) -> (→"Current Scan linear":cluster{dbl[], dbl[]})  [unwired: 1 out]
                  n163 = Bundle(w292, w298) -> (→"Current Scan log":cluster{dbl[], dbl[]})  [unwired: 1 out]
                  n164 = local read "Measured Vds"() -> (w304:dbl)
                  n165 = local read "Measured Igs"() -> (w307:dbl)
                  n166 = Build Array (concatenate)(w303, w304) -> (w299:dbl[])
                  n167 = Build Array (concatenate)(w306, w307) -> (w294:dbl[])
                }
              }
            }
            n168 = Build Array (concatenate)(w175, w169) -> (w170:dbl[])
            n169 = Build Array (concatenate)(w162, w163) -> (w164:dbl[])
            n170 = Build Array (concatenate)(w167, w165) -> (w166:dbl[])
            n171 = Build Array (concatenate)(w172, w159) -> (w171:dbl[])
            n172 = Build Array (concatenate)(w174, w168) -> (w173:dbl[])
          }
        }
        n173 = Bundle(w123, w125) -> (w126:cluster{dbl[], dbl[]})  [unwired: 1 out]
        n174 = Bundle(w123, w125) -> (w124:cluster{dbl[], dbl[]})  [unwired: 1 out]
        n175 = Bundle(w123, w122) -> (w134:cluster{dbl[], dbl[]})  [unwired: 1 out]
        n176 = Bundle(w123, w122) -> (w121:cluster{dbl[], dbl[]})  [unwired: 1 out]
      }
      "?" <- w108
      "Igs array" <- w97
      "Vgs array" <- w109
      "Ids array" <- w111
      "Vds array" <- w110
      "corrected PD current array" <- w96
      "Ids array 2" <- w94
      "Corrected PD current array 2" <- w93
      "Vds array 2" <- w92
      "Vgs array 2" <- w91
      "Igs array 2" <- w90
      "?" <- w89
      "?" <- w87
      "?" <- w88
      n177 = Multiply(x=w78, y=sgl 5.0) -> (x*y=w79:sgl)
      n178 = Build Array(w84) -> (w85:T2)
      n179 = Resize Matrix(1:w79, 2:w81, 4:w85) -> (0:→"data matrix":T2)
    }
    frame #4 {
      w322 = 0 items=["Set", "Get"] ("Operation (0: Set)")
      w324 = 1 items=["Current", "Voltage"] ("Source Mode (1: Voltage)")
      w321 = 1 items=["Channel 1", "Channel 2"] ("Channel (0: Channel 1)")
      w325 = 1 items=["Pulse", "DC"] ("Source Shape (1: DC)")
      w330 = 0 items=["Set", "Get"] ("Operation (0: Set)")
      w332 = 1 items=["Current", "Voltage"] ("Source Mode (1: Voltage)")
      w329 = 0 items=["Channel 1", "Channel 2"] ("Channel (0: Channel 1)")
      w333 = 1 items=["Pulse", "DC"] ("Source Shape (1: DC)")
      n180 = local read "Agilent address out"() -> (w313:refnum<visa-resource-name>)
      n181 = local read "error out agilent"() -> (w312:errorcluster)
      n182 = local read "light emission ON/OFF"() -> (w337:bool)
      n183 = case shown="True" w337 {
        frame False {
        }
        frame True {
          # "Turn 6487  off"
          n184 = local read "keithley address out"() -> (w339:refnum<k15>)
          n185 = local read "error out keithley"() -> (w338:errorcluster)
          n186 = call <instrlib>:"KE6485 Close.vi"("error in (no error)"=w338, "instrument handle"=w339) -> ("error out"=w340:errorcluster)  [unwired: 9 out]
          n187 = local write "error out keithley"(w340) -> ()
        }
      }
      n188 = call <instrlib>:"Configure Source.vi"("VISA resource name"=w313, "Channel (0: Channel 1)"=w329, "error in (no error)"=w312, "Source Shape (1: DC)"=w333, "Source Mode (1: Voltage)"=w332, "Output Level (0)"=0.0) -> ("VISA resource name out"=w335:refnum<visa-resource-name>, "error out"=w331:errorcluster)  [unwired: 12 in]
      n189 = call <instrlib>:"Enable Output.vi"("Enable Output (T: Enable)"=FALSE, "error in (no error)"=w331, "Operation (0: Set)"=w330, "Channel (0: Channel 1)"=w329, "VISA resource name"=w335) -> ("error out"=w319:errorcluster, "Output Enabled?"=w315:bool, "VISA resource name out"=w320:refnum<visa-resource-name>)  [unwired: 4 in]
      n190 = local write "channel 1 status"(w315) -> ()
      n191 = call <instrlib>:"Configure Source.vi"("VISA resource name"=w320, "Channel (0: Channel 1)"=w321, "error in (no error)"=w319, "Source Shape (1: DC)"=w325, "Source Mode (1: Voltage)"=w324, "Output Level (0)"=0.0) -> ("VISA resource name out"=w327:refnum<visa-resource-name>, "error out"=w323:errorcluster)  [unwired: 12 in]
      n192 = call <instrlib>:"Enable Output.vi"("Enable Output (T: Enable)"=FALSE, "error in (no error)"=w323, "Operation (0: Set)"=w322, "Channel (0: Channel 1)"=w321, "VISA resource name"=w327) -> ("error out"=w318:errorcluster, "Output Enabled?"=w316:bool, "VISA resource name out"=w317:refnum<visa-resource-name>)  [unwired: 4 in]
      n193 = local write "channel 2 status"(w316) -> ()
      n194 = call <instrlib>:"Close.vi"("error in (no error)"=w318, "VISA resource name"=w317) -> ("error out"=w314:errorcluster)  [unwired: 9 in]
      n195 = local write "error out agilent"(w314) -> ()
    }
    frame #5 {
      n196 = local read "corrected PD current array"() -> (w342:dbl[])
      n197 = local read "Vgs array"() -> (w341:dbl[])
      n198 = local read "Vgs array"() -> (w344:dbl[])
      n199 = local read "Ids array"() -> (w345:dbl[])
      n200 = local read "Igs array"() -> (w343:dbl[])
      n201 = Two Button Dialog(message="Do you want to save the data?") -> (T button?=w346:bool)  [unwired: 2 out]
      n202 = case shown="True" w346 {
        tunnel: w344 -> [_ w353]
        tunnel: w345 -> [_ w352]
        tunnel: w343 -> [_ w350]
        tunnel: w342 -> [_ w349]
        tunnel: w341 -> [_ w351]
        frame False {
        }
        frame True {
          n203 = Build Array(w351, w352, w353, w350, w349) -> ()  [unwired: 1 out]
          n204 = local read "data matrix"() -> (w348:dbl[][])
          n205 = call-poly <vilib>:"Write To Spreadsheet File.vi"("transpose? (no:F)"=FALSE, "format (%.3f)"="%.4e", "append to file? (new file:F)"=FALSE, "2D data"=w348) -> ()  [unwired: 4 in, 1 out]
        }
      }
    }
  }
